vi "nanocal -- nuclear schottky fit V5.vi"() -> ()   [LabVIEW 2020] (continued)
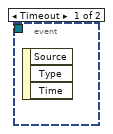
[diagram p2: hidden frame]
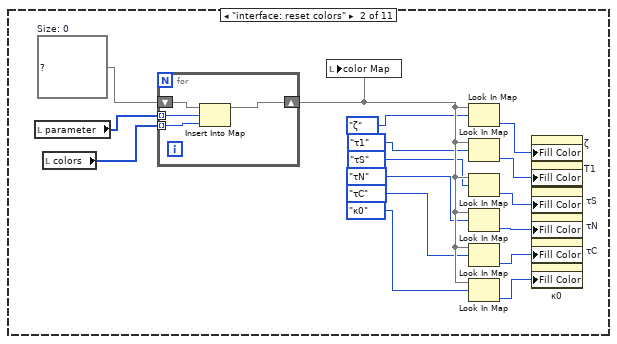
[diagram p4: hidden frame]
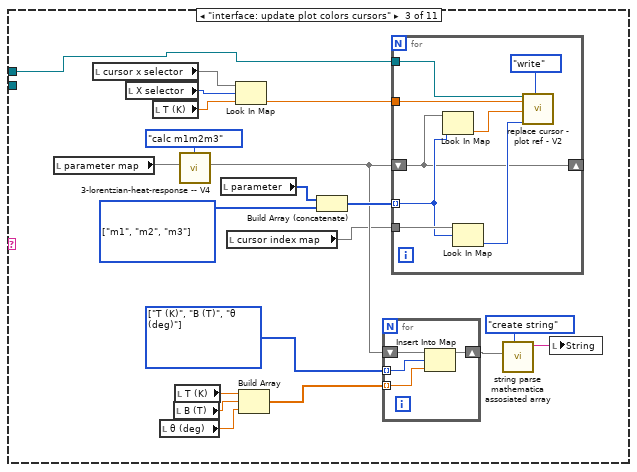
[diagram p5: hidden frame]
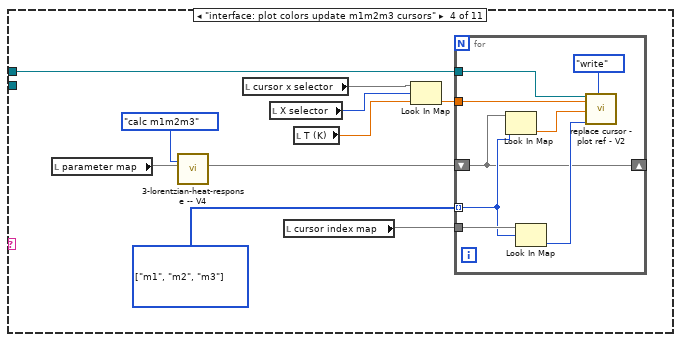
[diagram p6: hidden frame]
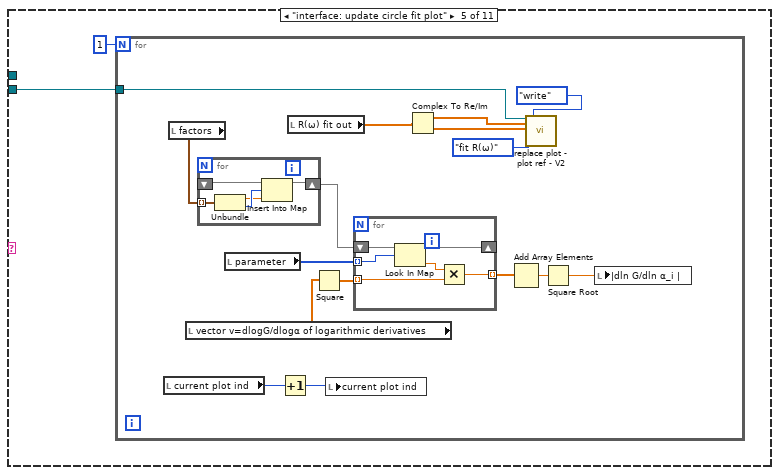
[diagram p7: hidden frame]
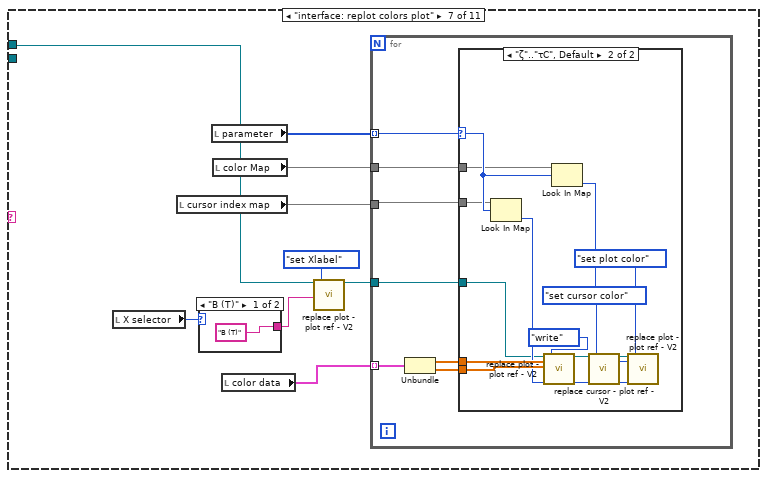
[diagram p9: hidden frame]
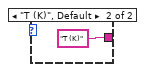
[diagram p10: hidden frame]
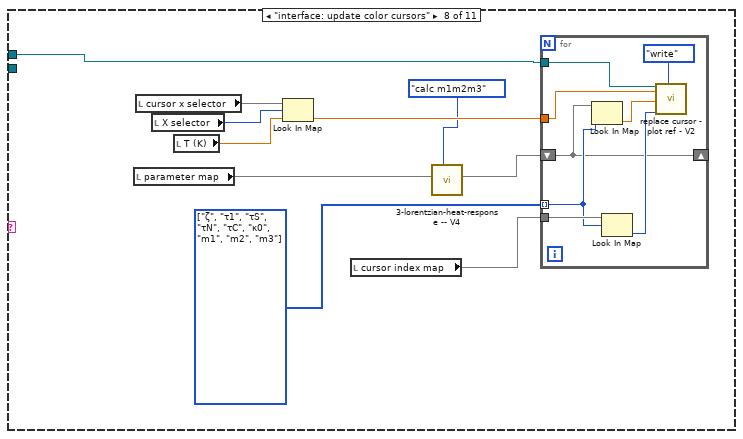
[diagram p12: hidden frame]
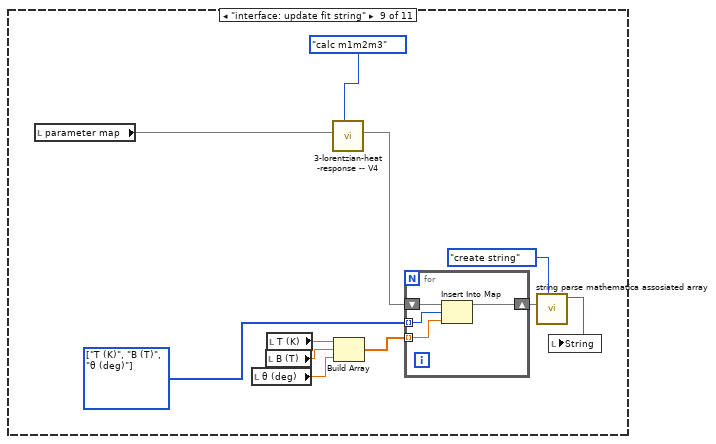
[diagram p13: hidden frame]
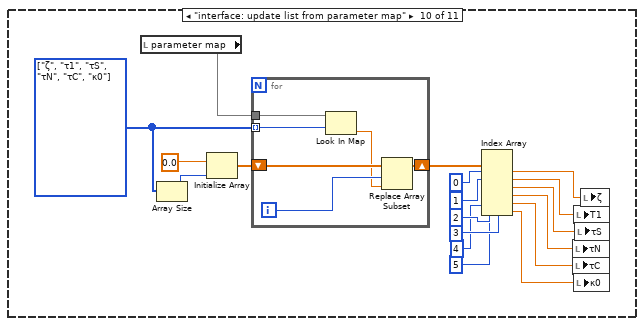
[diagram p14: hidden frame]
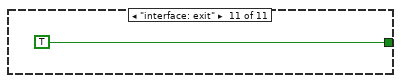
[diagram p15: hidden frame]
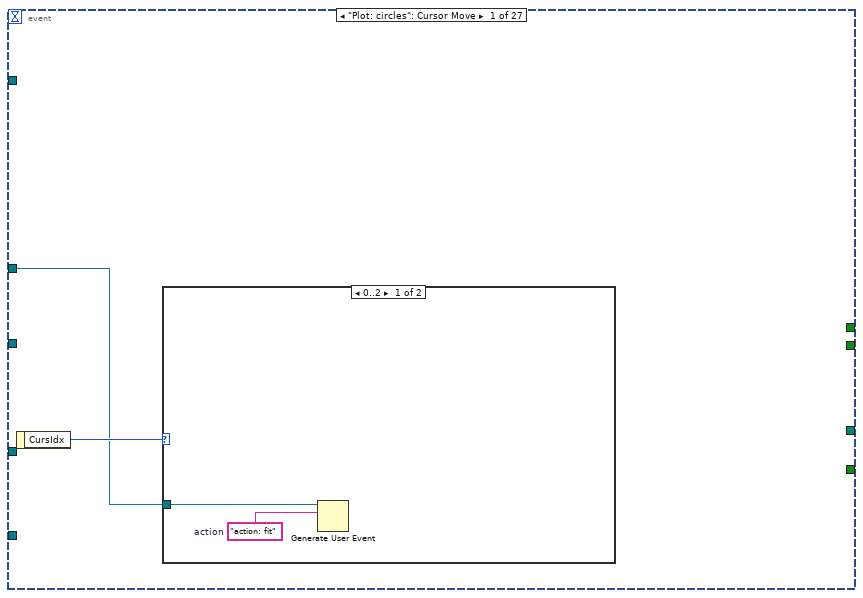
[diagram p16: hidden frame]
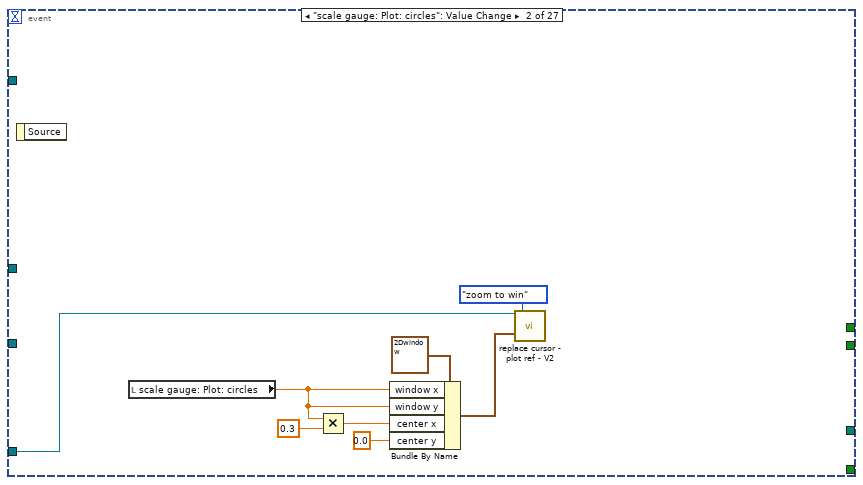
[diagram p18: hidden frame]
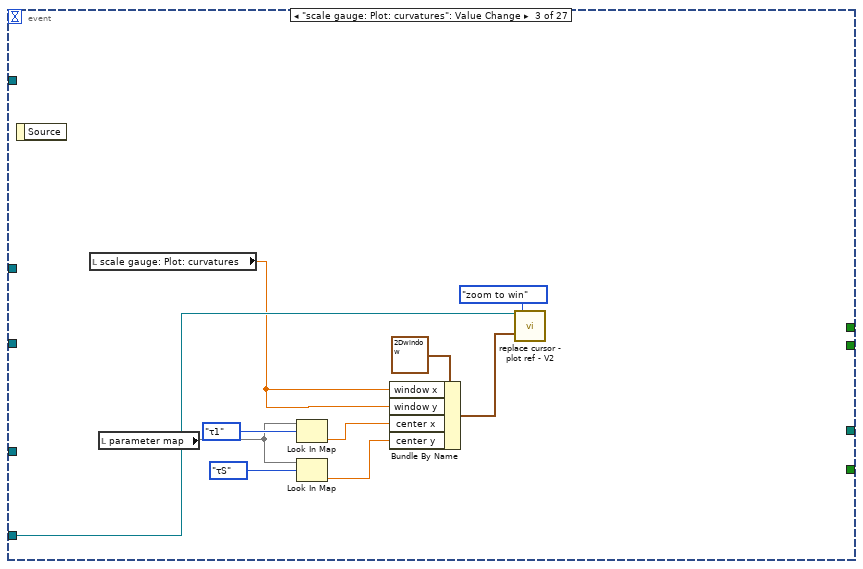
[diagram p19: hidden frame]
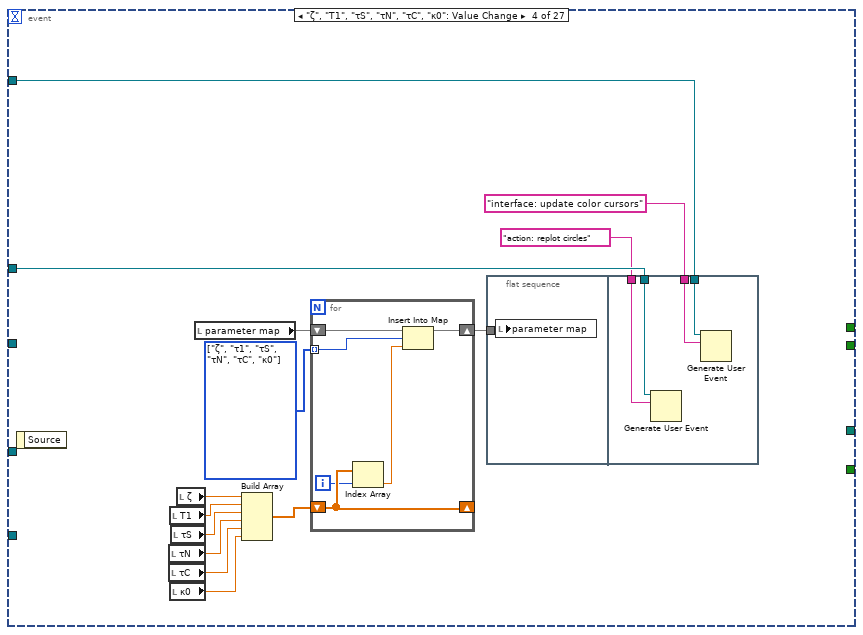
[diagram p20: hidden frame]
            n616 = call "3-lorentzian-heat-response -- V4.vi"("action"=3-lorentzian-heat-response_action."calc m1m2m3", "Map IN"=w1253) -> ("Map OUT"=w1260:map{T4, dbl})  [unwired: 7 in, 2 out]
            n617 = Build Array(w1257, w1258, w1259) -> (w1261:dbl[])
            n618 = for {
              shift-right: [w1266] -> w1262
              shift-left: w1260 -> [w1267]
              tunnel: w1255 -> [w1265] mode=indexing
              tunnel: w1261 -> [w1264] mode=indexing
              n619 = Insert Into Map(map in=w1267, key=w1265, value=w1264) -> (map out=w1266:map{T4, dbl})  [unwired: 2 out]
            }
            n620 = call "string parse mathematica assosiated array.vi"("action"=mathematica_string_map_action."create string" ("derivative"), "map IN"=w1262) -> ("String OUT"=w1263:string)  [unwired: 8 in, 1 out]
            n621 = local write "String"(w1263) -> ()
          }
          frame "interface: update list from parameter map" {
            w1269 = T4[] [enum."ζ", enum."τ1", enum."τS", enum."τN", enum."τC", enum."κ0"] items=["ζ", "τ1", "τS", "τN", "τC", "κ0", "m1", "m2", "m3", "T (K)", "B (T)", "θ (deg)", "side (S|R)", "set of (B|T)", "Re(offset)", "Im(offset)"]
            n622 = local read "parameter map"() -> (w1272:map{T4, dbl})
            n623 = Array Size(array=w1269) -> (size(s)=w1268:i32)
            n624 = Initialize Array(0.0 ("new X"), w1268) -> (w1271:dbl[])
            n625 = for {
              tunnel: w1269 -> [w1290] mode=indexing
              tunnel: w1272 -> [w1291]
              shift-right: [w1288] -> w1274
              shift-left: w1271 -> [w1289]
              i -> [w1287]
              n626 = Look In Map(map=w1291, key=w1290) -> (value=w1286:dbl)  [unwired: 1 in, 1 out]
              n627 = Replace Array Subset(array=w1289, new element=w1286, index=w1287) -> (w1288:dbl[])
            }
            n628 = Index Array(array=w1274, index #1=0 ("index"), index #2=1 ("index"), index #3=2 ("index"), index #4=3 ("index"), index #5=4 ("index"), index #6=5 ("index")) -> (element #1=w1273:dbl, element #2=w1281:dbl, element #3=w1282:dbl, element #4=w1283:dbl, element #5=w1284:dbl, element #6=w1285:dbl)
            n629 = local write "τN"(w1283) -> ()
            n630 = local write "τC"(w1284) -> ()
            n631 = local write "T1"(w1281) -> ()
            n632 = local write "κ0"(w1285) -> ()
            n633 = local write "τS"(w1282) -> ()
            n634 = local write "ζ"(w1273) -> ()
          }
          frame "interface: exit" {
          }
        }
      }
    }
  }
  n635 = while "interface" {
    tunnel: w7 -> [w1298]
    tunnel: w36 -> [w1297]
    tunnel: w33 -> [w1296]
    tunnel: w8 -> [w1295]
    tunnel: w1 -> [w1293]
    stop <- FALSE stop-if-true
    n636 = event shown="[14] Key Down" {
      selector: _ -> [_ _ _ _ _ _ _ _ _ _ _ _ _ _ _ _ _ _ _ _ _ _ _ _ _ _ _]
      dyn-events: _ -> [_ _ _ _ _ _ _ _ _ _ _ _ _ _ _ _ _ _ _ _ _ _ _ _ _ _ _]
      timeout: _ -> [_ _ _ _ _ _ _ _ _ _ _ _ _ _ _ _ _ _ _ _ _ _ _ _ _ _ _]
      tunnel: w1298 -> [w1299 _ _ w1322 w1346 _ w1371 w1377 _ w1381 w1383 w1385 w1387 w1390 w1397 w1492 w1513 w1533 w1535 w1539 w1542 w1545 w1548 w1556 w1560 w1562 w1565]
      tunnel: [_ _ _ _ _ _ _ _ _ "load! :l" _ _ _ _ _ _ _ _ _ _ _ _ _ _ _ _ _] -> _
      tunnel: [_ _ _ _ _ _ "go / pause!" _ _ _ _ _ _ "parse! :p" _ _ _ "Math→τ! :q" _ "τ→Math! :p" "Math→ string OUT! :s" "generate empty string from filelist !" "string IN → Math!" _ _ "plot landscape!" _] -> _
      tunnel: w1297 -> [_ w1303 _ _ _ w1348 _ _ _ _ _ _ _ _ w1393 _ _ _ _ _ _ _ _ _ _ _ _]
      tunnel: w1296 -> [_ _ _ _ _ _ _ _ _ _ _ _ _ _ _ w1500 w1521 _ _ _ _ _ _ _ _ _ _]
      tunnel: [_ _ _ _ _ _ _ _ _ _ "Read from file" _ _ _ _ _ _ _ _ _ _ _ _ _ _ _ _] -> _
      tunnel: [_ _ _ _ _ _ _ _ _ _ _ _ _ _ _ _ _ _ "load default values" _ _ _ _ _ _ _ _] -> _
      tunnel: w1295 -> [_ _ _ w1324 _ _ _ _ _ _ _ _ _ _ _ w1490 w1511 _ _ _ _ _ _ _ _ _ _]
      tunnel: w1293 -> [_ _ w1317 _ _ _ _ _ _ _ _ _ _ _ w1392 _ _ _ _ _ _ _ _ _ _ _ _]
      event "Plot: circles": Cursor Move {
        n637 = event-data() -> ("CursIdx"=w1300:i32)  [unwired: 1 in]
        n638 = case shown="0..2" w1300 {
          tunnel: w1299 -> [w1302 _]
          frame 0..2 {
            w1301 = "action: fit"  # action
            n639 = Generate User Event(user event=w1302, event data cluster=w1301) -> ()  [unwired: 2 in, 2 out]
          }
          frame 3..5, Default {
          }
        }
      }
      event "scale gauge: Plot: circles": Value Change {
        n640 = event-data() -> ()  [unwired: 1 in, 1 out]
        n641 = local read "scale gauge: Plot: circles"() -> (w1309:dbl)
        n642 = Multiply(x=w1309, y=0.3) -> (x*y=w1310:dbl)
        n643 = Bundle By Name(cluster=T36 {"window y"=0.0021014740628288917, "center x"=44850.89441339177, "center y"=2.5658109925320947, "window x"=17480.201988350764} ("window IN"), "window x"=w1309, "window y"=w1309, "center x"=w1310, "center y"=0.0) -> (w1308:T36)
        n644 = call "replace cursor - plot ref - V2.vi"("Plot ref in"=w1303, "window IN"=w1308, "cursor action"=cursor_action."zoom to win") -> ()  [unwired: 13 in, 4 out]
      }
      event "scale gauge: Plot: curvatures": Value Change {
        n645 = event-data() -> ()  [unwired: 1 in, 1 out]
        n646 = local read "scale gauge: Plot: curvatures"() -> (w1313:dbl)
        n647 = local read "parameter map"() -> (w1314:map{T4, dbl})
        n648 = Look In Map(map=w1314, key=3-lorentzian-parameters."τ1") -> (value=w1312:dbl)  [unwired: 1 in, 1 out]
        n649 = Look In Map(map=w1314, key=3-lorentzian-parameters."τS") -> (value=w1311:dbl)  [unwired: 1 in, 1 out]
        n650 = Bundle By Name(cluster=T36 {"window y"=0.0021014740628288917, "center x"=44850.89441339177, "center y"=2.5658109925320947, "window x"=17480.201988350764} ("window IN"), "window x"=w1313, "window y"=w1313, "center x"=w1312, "center y"=w1311) -> (w1320:T36)
        n651 = call "replace cursor - plot ref - V2.vi"("Plot ref in"=w1317, "window IN"=w1320, "cursor action"=cursor_action."zoom to win") -> ()  [unwired: 13 in, 4 out]
      }
      event "ζ", "T1", "τS", "τN", "τC", "κ0": Value Change {
        w1325 = T4[] [enum."ζ", enum."τ1", enum."τS", enum."τN", enum."τC", enum."κ0"] items=["ζ", "τ1", "τS", "τN", "τC", "κ0", "m1", "m2", "m3", "T (K)", "B (T)", "θ (deg)", "side (S|R)", "set of (B|T)", "Re(offset)", "Im(offset)"]
        n652 = event-data() -> ()  [unwired: 1 in, 1 out]
        n653 = local read "τN"() -> (w1331:dbl)
        n654 = local read "τC"() -> (w1330:dbl)
        n655 = local read "T1"() -> (w1333:dbl)
        n656 = local read "κ0"() -> (w1329:dbl)
        n657 = local read "τS"() -> (w1332:dbl)
        n658 = local read "ζ"() -> (w1334:dbl)
        n659 = local read "parameter map"() -> (w1326:map{T4, dbl})
        n660 = Build Array(w1334, w1333, w1332, w1331, w1330, w1329) -> (w1328:dbl[])
        n661 = for {
          tunnel: w1325 -> [w1340] mode=indexing
          shift-right: [w1345] -> _
          shift-left: w1328 -> [w1345]
          shift-right: [w1342] -> w1327
          shift-left: w1326 -> [w1343]
          i -> [w1344]
          n662 = Index Array(array=w1345, index=w1344) -> (element=w1341:dbl)
          n663 = Insert Into Map(map in=w1343, key=w1340, value=w1341) -> (map out=w1342:map{T4, dbl})  [unwired: 2 out]
        }
        n664 = flat-sequence {
          tunnel: w1327 -> [w1335]
          tunnel: w1324 -> [w1339]
          tunnel: "interface: update color cursors" ("event data") -> [w1338]
          tunnel: w1322 -> [w1337]
          tunnel: "action: replot circles" ("event data") -> [w1336]
          frame #0 {
            n665 = local write "parameter map"(w1335) -> ()
          }
          frame #1 {
            n666 = Generate User Event(user event=w1337, event data cluster=w1336) -> ()  [unwired: 2 in, 2 out]
            n667 = Generate User Event(user event=w1339, event data cluster=w1338) -> ()  [unwired: 2 in, 2 out]
          }
        }
      }
      event Value Change {
        n668 = event-data() -> ()  [unwired: 1 in, 6 out]
        n669 = Generate User Event(user event=w1346, event data cluster="action: update enums" ("event data")) -> ()  [unwired: 2 in, 2 out]
      }
      event "ω0 (rad/sec)": Value Change {
        n670 = event-data() -> ()  [unwired: 1 in, 1 out]
        n671 = local read "parameter map"() -> (w1350:map{T4, dbl})
        n672 = call "nanocal -- publish -- freq scan V2.vi"("publisher action"=publisher_action."get") -> ("z out (V)"=w1368:cdb[], "ω out (Hz)"=w1363:dbl[])  [unwired: 7 in, 2 out]
        n673 = Divide(x="ω0 (rad/sec)", y=6.283185307179586) -> (x/y=w1361:dbl)
        n674 = call "3-lorentzian-heat-response -- V4.vi"("action"=3-lorentzian-heat-response_action."calc R", "Map IN"=w1350, "omega IN (rad/sec)"="ω0 (rad/sec)") -> ("Romega"=w1360:cdb)  [unwired: 6 in, 2 out]
        n675 = Threshold 1D Array(2:w1361, 3:w1363) -> (0:w1362:dbl)  [unwired: 1 in]
        n676 = Complex To Re/Im(x + iy=w1360) -> (x=w1358:dbl, y=w1359:dbl)
        n677 = Index Array(array=w1368, index=w1362) -> (element=w1365:cdb)
        n678 = call "replace cursor - plot ref - V2.vi"("Plot ref in"=w1348, "new X"=w1358, "new  Y"=w1359, "cursor index"=0, "cursor action"=cursor_action."write") -> ("Plot ref out"=w1364:refnum<vi>)  [unwired: 11 in, 3 out]
        n679 = Complex To Re/Im(x + iy=w1365) -> (x=w1366:dbl, y=w1367:dbl)
        n680 = call "replace cursor - plot ref - V2.vi"("Plot ref in"=w1364, "new X"=w1366, "new  Y"=w1367, "cursor index"=1, "cursor action"=cursor_action."write") -> ()  [unwired: 11 in, 4 out]
      }
      event "go / pause!": Value Change {
        n681 = event-data() -> ()  [unwired: 1 in, 1 out]
        n682 = local read "newton is active"() -> (w1369:bool)
        n683 = case shown="True" w1369 {
          tunnel: w1371 -> [_ w1376]
          tunnel: [FALSE TRUE] -> w1370
          frame True {
          }
          frame False {
            n684 = Generate User Event(user event=w1376, event data cluster="action: gradient step" ("event data")) -> ()  [unwired: 2 in, 2 out]
          }
        }
        n685 = local write "newton is active"(w1370) -> ()
      }
      event "selector": Value Change {
        n686 = event-data() -> ()  [unwired: 1 in, 1 out]
        n687 = Generate User Event(user event=w1377, event data cluster="action: update state of selectors" ("event data")) -> ()  [unwired: 2 in, 2 out]
      }
      event "Plot: circles": Cursor Release {
        n688 = event-data() -> ()  [unwired: 1 in, 1 out]
      }
      event "load! :l": Value Change {
        n689 = event-data() -> ()  [unwired: 1 in, 6 out]
        n690 = Generate User Event "action User Event"(user event=w1381, event data cluster="action: read from file" ("event data")) -> ()  [unwired: 2 in, 2 out]
      }
      event "Read from file": Value Change {
        n691 = event-data() -> ()  [unwired: 1 in, 6 out]
        n692 = Generate User Event ("action User Event")(user event=w1383, event data cluster="action: read from file" ("event data")) -> ()  [unwired: 2 in, 2 out]
      }
      event "offset Re\noffset Im": Value Change {
        n693 = event-data() -> ()  [unwired: 1 in, 6 out]
        n694 = Generate User Event "action User Event"(user event=w1385, event data cluster="action: read from file" ("event data")) -> ()  [unwired: 2 in, 2 out]
      }
      event "cspan": Value Change {
        n695 = event-data() -> ()  [unwired: 1 in, 6 out]
        n696 = Generate User Event "action User Event"(user event=w1387, event data cluster="action: read from file" ("event data")) -> ()  [unwired: 2 in, 2 out]
      }
      event "parse! :p": Value Change {
        n697 = event-data() -> ()  [unwired: 1 in, 6 out]
        n698 = Generate User Event "action User Event"(user event=w1390, event data cluster="action: parse string" ("event data")) -> ()  [unwired: 2 in, 2 out]
      }
      event Key Down {
        n699 = event-data() -> ("Char"=w1395:i16, "VKey"=w1398:T37)  [unwired: 1 in]
        n700 = Build Array(w1395) -> (w1396:i16[])
        n701 = Byte Array To String(unsigned byte array=w1396) -> (string=w1394:string)
        n702 = case shown="\"ASCII\", Default" w1398 {
          selector: w1398 -> [_ _ _ _ _ w1483]
          tunnel: w1397 -> [w1402 _ w1478 _ _ _]
          tunnel: w1394 -> [w1401 _ _ _ _ _]
          tunnel: w1393 -> [w1400 _ _ _ _ w1482]
          tunnel: w1392 -> [w1399 _ _ _ _ _]
          frame "ASCII", Default {
            n703 = case shown="\"?\"" w1401 {
              selector: w1401 -> [_ _ _ _ _ _ w1427 w1437 _ _ _ _ w1457 _]
              tunnel: w1402 -> [_ _ w1403 w1405 w1409 _ _ _ _ w1448 w1451 w1453 w1455 w1476]
              tunnel: w1400 -> [_ _ _ _ _ w1423 _ _ _ _ _ _ _ _]
              tunnel: w1399 -> [_ _ _ _ _ w1416 _ _ _ _ _ _ _ _]
              frame "0", Default {
              }
              frame "a" {
              }
              frame "s" {
                n704 = Generate User Event(user event=w1403, event data cluster="action: write mathematica string" ("event data")) -> ()  [unwired: 2 in, 2 out]
              }
              frame "l" {
                n705 = Generate User Event(user event=w1405, event data cluster="action: read from file" ("event data")) -> ()  [unwired: 2 in, 2 out]
              }
              frame " " {
                n706 = local read "newton is active"() -> (w1408:bool)
                n707 = case shown="False" w1408 {
                  selector: w1408 -> [w1411 w1413]
                  tunnel: w1409 -> [_ w1415]
                  tunnel: [w1410 w1412] -> w1407
                  frame True {
                    n708 = Not(x=w1411) -> (.not. x?=w1410:bool)
                  }
                  frame False {
                    n709 = Generate User Event(user event=w1415, event data cluster="action: gradient step" ("event data")) -> ()  [unwired: 2 in, 2 out]
                    n710 = Not(x=w1413) -> (.not. x?=w1412:bool)
                  }
                }
                n711 = local write "newton is active"(w1407) -> ()
              }
              frame "?" {
                # "?"
                n712 = call "replace cursor - plot ref - V2.vi"("Plot ref in"=w1423, "cursor action"=cursor_action."zoom to win") -> ("Plot ref out"=w1422:refnum<vi>)  [unwired: 14 in, 3 out]
                n713 = call "replace cursor - plot ref - V2.vi"("Plot ref in"=w1422, "cursor action"=cursor_action."smart zoom out&aspect") -> ()  [unwired: 14 in, 4 out]
                n714 = call "replace cursor - plot ref - V2.vi"("Plot ref in"=w1416, "cursor action"=cursor_action."zoom to win") -> ("Plot ref out"=w1419:refnum<vi>)  [unwired: 14 in, 3 out]
                n715 = call "replace cursor - plot ref - V2.vi"("Plot ref in"=w1419, "cursor action"=cursor_action."smart zoom out&aspect") -> ()  [unwired: 14 in, 4 out]
              }
              frame ",", "." {
                n716 = local read "newton parameters"() -> (w1425:T5)
                n717 = case shown="\".\"" w1427 {
                  tunnel: [0.7 1.0 1.5] -> w1426
                  frame "," {
                  }
                  frame "0", Default {
                  }
                  frame "." {
                  }
                }
                n718 = in-place {
                  in-place-border: w1426 -> [w1430]
                  n719 = in-place-cluster #7(w1425) -> ("PID-P"=w1428:dbl)
                  n720 = Multiply(x=w1430, y=w1428) -> (x*y=w1429:dbl)
                  n721 = in-place-cluster #7("PID-P"=w1429) -> (w1424:T5)
                }
                n722 = local write "newton parameters"(w1424) -> ()
              }
              frame "<", ">" {
                n723 = local read "newton parameters"() -> (w1435:T5)
                n724 = case shown="\"<\"" w1437 {
                  tunnel: [-5 0 5] -> w1436
                  frame "<" {
                  }
                  frame "0", Default {
                  }
                  frame ">" {
                  }
                }
                n725 = in-place {
                  in-place-border: w1436 -> [w1443]
                  n726 = in-place-cluster #8(w1435) -> ("PID-I"=w1442:i32)
                  n727 = Add(x=w1443, y=w1442) -> (x+y=w1441:i32)
                  n728 = In Range and Coerce(upper limit=100, x=w1441, lower limit=2) -> (coerced(x)=w1438:i32)  [unwired: 1 out]
                  n729 = in-place-cluster #8("PID-I"=w1438) -> (w1434:T5)
                }
                n730 = local write "newton parameters"(w1434) -> ()
              }
              frame "b" {
                n731 = local read "String"() -> (w1447:string)
                n732 = local write "backup string :b"(w1447) -> ()
              }
              frame "u" {
                n733 = Generate User Event(user event=w1448, event data cluster="ignoreaction: uco" ("event data")) -> ()  [unwired: 2 in, 2 out]
              }
              frame "p" {
                n734 = Generate User Event "action User Event"(user event=w1451, event data cluster="action: copy to math" ("event data")) -> ()  [unwired: 2 in, 2 out]
              }
              frame "q" {
                n735 = Generate User Event "action User Event"(user event=w1453, event data cluster="action: copy from math" ("event data")) -> ()  [unwired: 2 in, 2 out]
              }
              frame "\\", "|" {
                n736 = for {
                  N: 1 -> [_]
                  tunnel: w1457 -> [w1471]
                  tunnel: w1455 -> [w1470]
                  tunnel: [w1470] -> w1454
                  n737 = local read "selection :|\\"() -> (w1463:u16)
                  n738 = property on="selection :|\\" class="Ring (strict)"() -> ("NumItems"=w1461:u32)  [unwired: 2 in, 2 out]
                  n739 = To Long Integer(number=w1463) -> (32bit integer=w1462:i32)
                  n740 = case shown="\"|\", Default" w1471 {
                    tunnel: w1462 -> [w1473 w1475]
                    tunnel: [w1472 w1474] -> w1467
                    frame "|", Default {
                      n741 = Decrement(x=w1473) -> (x-1=w1472:i32)
                    }
                    frame "\\" {
                      n742 = Increment(x=w1475) -> (x+1=w1474:i32)
                    }
                  }
                  n743 = To Long Integer(number=w1461) -> (32bit integer=w1460:i32)
                  n744 = Greater Or Equal?(x=w1467, y=w1460) -> (x >= y?=w1469:bool)
                  n745 = Select(t=u16 0 ("lower limit"), s=w1469, f=w1467) -> (s? t:f=w1464:i32)
                  n746 = Decrement(x=w1460) -> (x-1=w1465:i32)
                  n747 = Less Than 0?(x=w1464) -> (x < 0?=w1466:bool)
                  n748 = Select(t=w1465, s=w1466, f=w1464) -> (s? t:f=w1459:i32)
                  n749 = local write "selection :|\\"(w1459) -> ()
                }
                n750 = Generate User Event ("action User Event")(user event=w1454, event data cluster="action: constrained filenames select" ("event data")) -> ()  [unwired: 2 in, 2 out]
              }
              frame "m" {
                n751 = Generate User Event "action User Event"(user event=w1476, event data cluster="action: copy from math" ("event data")) -> ()  [unwired: 2 in, 2 out]
              }
            }
          }
          frame "PageUp" {
          }
          frame "Enter" {
            n752 = Generate User Event ("action User Event")(user event=w1478, event data cluster="action: new sweep" ("event data")) -> (user event out=w1479:refnum<user-event>)  [unwired: 2 in, 1 out]
            n753 = Generate User Event ("action User Event")(user event=w1479, event data cluster="action: replot colors" ("event data")) -> ()  [unwired: 2 in, 2 out]
          }
          frame "Caps" {
          }
          frame "PageDown" {
          }
          frame "Up".."Right" {
            n754 = case shown="\"Down\"" w1483 {
              tunnel: [cursor_action."zoom in 20%" ("cursor action") cursor_action."zoom out 20%" ("cursor action") cursor_action."zoom out 20%" ("cursor action") cursor_action."zoom in 20%" ("cursor action")] -> w1484
              frame "Up", Default {
              }
              frame "Down" {
              }
              frame "Left" {
              }
              frame "Right" {
              }
            }
            n755 = call "replace cursor - plot ref - V2.vi"("Plot ref in"=w1482, "cursor action"=w1484) -> ()  [unwired: 14 in, 4 out]
          }
        }
      }
      event "Plot:  colors": Cursor Move {
        (unwired) "interface: plot colors update m1m2m3 cursors" ("event data")
        n756 = event-data() -> ("CursIdx"=w1498:i32)  [unwired: 1 in]
        n757 = local read "reverse cursor index map"() -> (w1499:map{i32, T4})
        n758 = call "replace cursor - plot ref - V2.vi"("Plot ref in"=w1500, "cursor index"=w1498, "cursor action"=cursor_action."read") -> ("read Y"=w1497:dbl)  [unwired: 13 in, 3 out]
        n759 = local read "parameter map"() -> (w1496:map{T4, dbl})
        n760 = Look In Map(map=w1499, key=w1498) -> (value=w1494:T4)  [unwired: 1 in, 1 out]
        n761 = in-place {
          in-place-border: w1497 -> [w1508]
          in-place-border: LVMapReplaceAction."Modify Entry only if found" ("action") -> [w1507]
          n762 = in-place-map #9(w1496, w1494) -> ()  [unwired: 1 in, 2 out]
          n763 = in-place-map #9(w1508, w1507) -> (w1495:map{T4, dbl})  [unwired: 2 out]
        }
        n764 = flat-sequence {
          tunnel: w1495 -> [w1502]
          tunnel: w1492 -> [w1506]
          tunnel: "action: replot circles" ("event data") -> [w1505]
          tunnel: w1490 -> [w1504]
          tunnel: "interface: update list from parameter map" ("event data") -> [w1503]
          frame #0 {
            n765 = local write "parameter map"(w1502) -> ()
          }
          frame #1 {
            n766 = Generate User Event(user event=w1506, event data cluster=w1505) -> ()  [unwired: 2 in, 2 out]
            n767 = Generate User Event(user event=w1504, event data cluster=w1503) -> ()  [unwired: 2 in, 2 out]
          }
        }
      }
      event "Plot:  colors": Cursor Release {
        n768 = event-data() -> ("CursIdx"=w1519:i32)  [unwired: 1 in]
        n769 = local read "reverse cursor index map"() -> (w1520:map{i32, T4})
        n770 = call "replace cursor - plot ref - V2.vi"("Plot ref in"=w1521, "cursor index"=w1519, "cursor action"=cursor_action."read") -> ("read Y"=w1518:dbl)  [unwired: 13 in, 3 out]
        n771 = local read "parameter map"() -> (w1517:map{T4, dbl})
        n772 = Look In Map(map=w1520, key=w1519) -> (value=w1515:T4)  [unwired: 1 in, 1 out]
        n773 = in-place {
          in-place-border: w1518 -> [w1531]
          in-place-border: LVMapReplaceAction."Modify Entry only if found" ("action") -> [w1530]
          n774 = in-place-map #10(w1517, w1515) -> ()  [unwired: 1 in, 2 out]
          n775 = in-place-map #10(w1531, w1530) -> (w1516:map{T4, dbl})  [unwired: 2 out]
        }
        n776 = flat-sequence {
          tunnel: w1516 -> [w1523]
          tunnel: w1513 -> [w1529]
          tunnel: "action: replot circles" ("event data") -> [w1528]
          tunnel: w1511 -> [w1527]
          tunnel: "interface: update list from parameter map" ("event data") -> [w1526]
          tunnel: "interface: plot colors update m1m2m3 cursors" ("event data") -> [w1524]
          frame #0 {
            n777 = local write "parameter map"(w1523) -> ()
          }
          frame #1 {
            n778 = Generate User Event(user event=w1529, event data cluster=w1528) -> ()  [unwired: 2 in, 2 out]
            n779 = Generate User Event(user event=w1527, event data cluster=w1526) -> (user event out=w1525:refnum<user-event>)  [unwired: 2 in, 1 out]
            n780 = Generate User Event(user event=w1525, event data cluster=w1524) -> ()  [unwired: 2 in, 2 out]
          }
        }
      }
      event "Math→τ! :q": Value Change {
        n781 = event-data() -> ()  [unwired: 1 in, 1 out]
        n782 = Generate User Event(user event=w1533, event data cluster="action: copy from math" ("event data")) -> ()  [unwired: 2 in, 2 out]
      }
      event "load default values": Value Change {
        n783 = event-data() -> ()  [unwired: 1 in, 1 out]
        n784 = Generate User Event(user event=w1535, event data cluster="action: update default values" ("event data")) -> ()  [unwired: 2 in, 2 out]
      }
      event "τ→Math! :p": Value Change {
        n785 = event-data() -> ()  [unwired: 1 in, 1 out]
        n786 = Generate User Event(user event=w1539, event data cluster="action: copy to math" ("event data")) -> ()  [unwired: 2 in, 2 out]
      }
      event "Math→ string OUT! :s": Value Change {
        n787 = event-data() -> ()  [unwired: 1 in, 1 out]
        n788 = Generate User Event(user event=w1542, event data cluster="action: write mathematica string" ("event data")) -> ()  [unwired: 2 in, 2 out]
      }
      event "generate empty string from filelist !": Value Change {
        n789 = event-data() -> ()  [unwired: 1 in, 1 out]
        n790 = Generate User Event(user event=w1545, event data cluster="action: empty string from filelist" ("event data")) -> ()  [unwired: 2 in, 2 out]
      }
      event "string IN → Math!": Value Change {
        n791 = event-data() -> ()  [unwired: 1 in, 1 out]
        n792 = Generate User Event(user event=w1548, event data cluster="action: read mathematica string" ("event data")) -> ()  [unwired: 2 in, 2 out]
      }
      event "filenames": Value Change {
        n793 = event-data() -> ()  [unwired: 1 in, 1 out]
        n794 = local read "filesnames lookup"() -> (w1555:map{i32, string})
        n795 = local read "all full filenames"() -> (w1553:map{string, path})
        n796 = local read "filenames"() -> (w1554:u16)
        n797 = Look In Map(map=w1555, key=w1554) -> (value=w1552:string)  [unwired: 1 in, 1 out]
        n798 = Look In Map(map=w1553, key=w1552) -> (value=w1550:path)  [unwired: 1 in, 1 out]
        n799 = for {
          N: 1 -> [_]
          tunnel: w1556 -> [w1558]
          tunnel: w1550 -> [w1557]
          n800 = local write "Read from file"(w1557) -> ()
          n801 = Generate User Event(user event=w1558, event data cluster="action: read from file" ("event data")) -> ()  [unwired: 2 in, 2 out]
        }
      }
      event "selection :|\\": Value Change {
        n802 = event-data() -> ()  [unwired: 1 in, 1 out]
        n803 = Generate User Event(user event=w1560, event data cluster="action: constrained filenames select" ("event data")) -> ()  [unwired: 2 in, 2 out]
      }
      event "plot landscape!", "range one", "range two": Value Change {
        n804 = event-data() -> ()  [unwired: 1 in, 6 out]
        n805 = Generate User Event(user event=w1562, event data cluster="action: plot landscape" ("event data")) -> ()  [unwired: 2 in, 2 out]
      }
      event "colors": Value Change {
        n806 = event-data() -> ()  [unwired: 1 in, 6 out]
        n807 = Generate User Event(user event=w1565, event data cluster="action: reset colors" ("event data")) -> ()  [unwired: 2 in, 2 out]
      }
    }
  }
  "cursor x selector" <- w34
